vi "test.vi"() -> (0 "picture":picture)   [LabVIEW 2013]
uses:
  <vilib>/Analysis/NI_AALBase.lvlib
panel:
  in  "Size":cluster{"horz":i16, "vert":i16}
  out "Red":T1(graph)
  out "Blue":T1(graph)
  out "Green":T1(graph)
  out "Intensity Graph":u8[][](graph)
  in  "Rectangle":cluster{"left":i16, "top":i16}
  in  "path to JPEG file":path
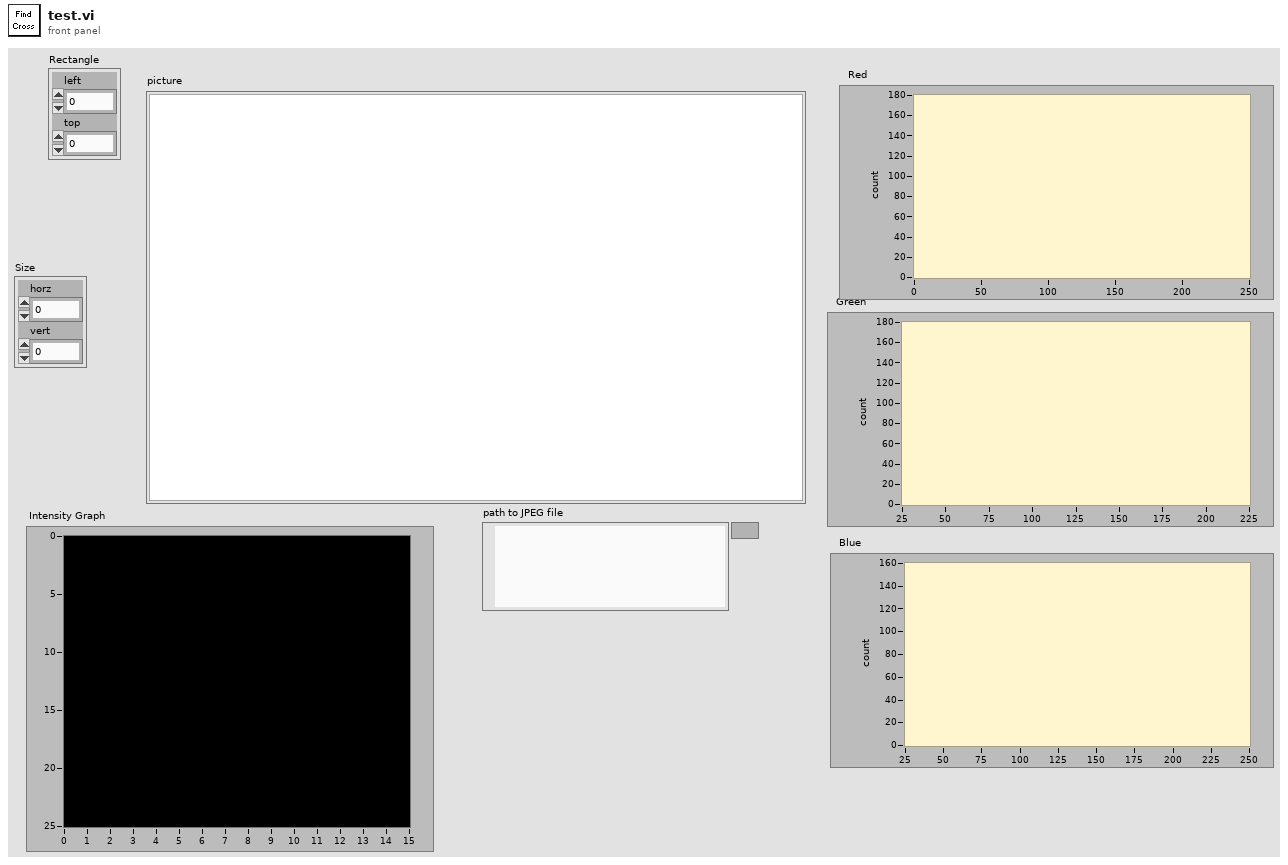
[diagram p1: front panel]
types:
  T1 = cluster{"X Values":dbl[], "Histogram: h(x)":i32[]}
  T2 = cluster{"left":i16, "top":i16, "right":i16, "bottom":i16}
  T3 = typedef "imagedata.ctl" = cluster{"image type":i32, "image depth":i32, "image":u8[], "mask":u8[], "colors":u32[], "Rectangle":cluster{"left":i16, "top":i16, "right":i16, "bottom":i16}}
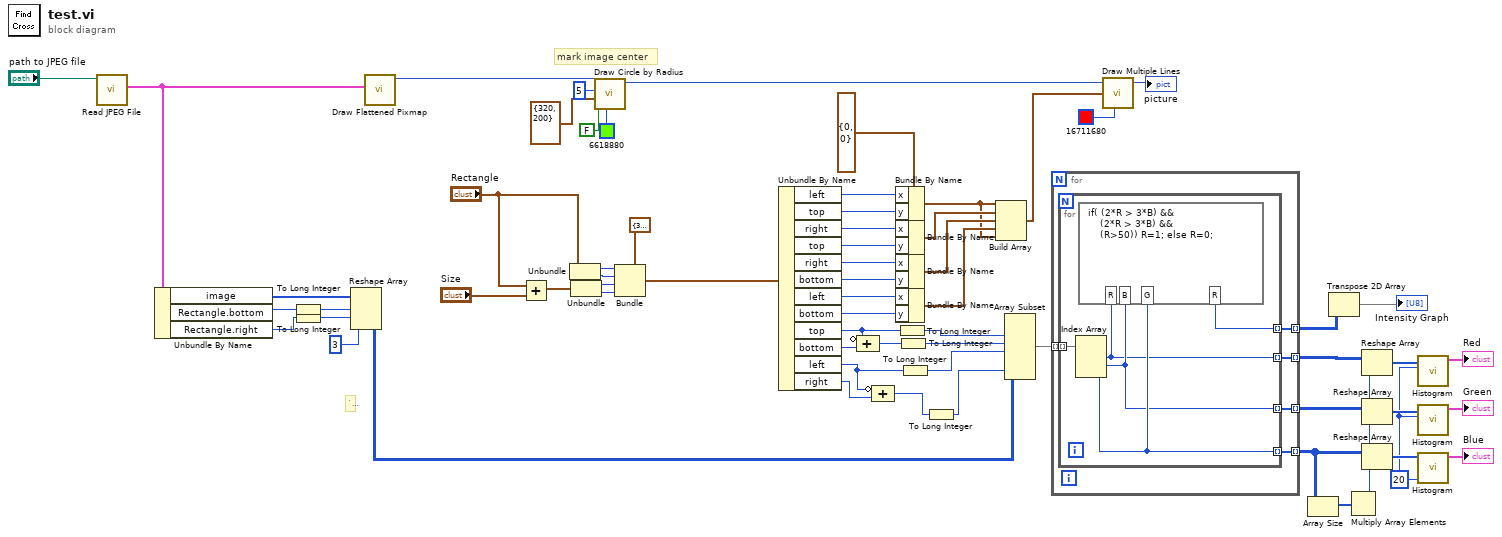
[diagram p0: block diagram]
diagram:
  w1 = 20 ("intervals")
  w55 = cluster{"x":i16, "y":i16} {"x"=0, "y"=0}
  # "``"
  # "mark image center"
  n1 = call <vilib>:"Read JPEG File.vi"("path to JPEG file"="path to JPEG file") -> ("image data"=w42:T3)  [unwired: 8 in, 2 out]
  n2 = Unbundle By Name(w42) -> ("image"=w41:u8[], "Rectangle.bottom"=w14:i16, "Rectangle.right"=w13:i16)
  n3 = To Long Integer(number=w14) -> (32bit integer=w12:i32)
  n4 = To Long Integer(number=w13) -> (32bit integer=w11:i32)
  n5 = Reshape Array(w41, w12, w11, 3 ("dimension size")) -> (w39:u8[][][])
  n6 = call <vilib>:"Draw Flattened Pixmap.vi"("image data"=w42) -> ("new picture"=w65:picture)  [unwired: 8 in]
  n7 = Add(x="Rectangle", y="Size") -> (x+y=w19:cluster{i16, i16})
  n8 = Unbundle("Rectangle") -> ("left"=w23:i16, "top"=w22:i16)
  n9 = Unbundle(w19) -> (w18:i16, w17:i16)
  n10 = call <vilib>:"Draw Circle by Radius.vi"("color(black)"=u32 6618880, "fill?(F)"=FALSE, "pixel center"=cluster{"horizontal":i16, "vertical":i16} {"horizontal"=320, "vertical"=200}, "radius"=i16 5, "picture"=w65) -> ("new picture"=w59:picture)  [unwired: 6 in]
  n11 = Bundle(cluster=T2 {"left"=300, "top"=100, "right"=400, "bottom"=200} ("Rectangle"), "left"=w23, "top"=w22, "right"=w18, "bottom"=w17) -> (w16:T2)
  n12 = Unbundle By Name(w16) -> ("left"=w57:i16, "top"=w56:i16, "right"=w54:i16, "top"=w53:i16, "right"=w52:i16, "bottom"=w51:i16, "left"=w50:i16, "bottom"=w49:i16, "top"=w8:i16, "bottom"=w9:i16, "left"=w7:i16, "right"=w6:i16)
  n13 = Compound Arithmetic op=ADD(invert w8, w9) -> (w37:i16)
  n14 = Compound Arithmetic op=ADD(invert w7, w6) -> (w5:i16)
  n15 = Bundle By Name(cluster=w55, "x"=w57, "y"=w56) -> (w43:cluster{"x":i16, "y":i16})
  n16 = Bundle By Name(cluster=w55, "x"=w54, "y"=w53) -> (w48:cluster{"x":i16, "y":i16})
  n17 = Bundle By Name(cluster=w55, "x"=w52, "y"=w51) -> (w47:cluster{"x":i16, "y":i16})
  n18 = Bundle By Name(cluster=w55, "x"=w50, "y"=w49) -> (w46:cluster{"x":i16, "y":i16})
  n19 = To Long Integer(number=w8) -> (32bit integer=w38:i32)
  n20 = To Long Integer(number=w37) -> (32bit integer=w36:i32)
  n21 = To Long Integer(number=w7) -> (32bit integer=w35:i32)
  n22 = To Long Integer(number=w5) -> (32bit integer=w4:i32)
  n23 = Build Array(w43, w48, w47, w46, w43) -> (w45:cluster{"x":i16, "y":i16}[])
  n24 = Array Subset(array=w39, index (dim 0)=w38, length (dim 0)=w36, index (dim 1)=w35, length (dim 1)=w4) -> (w34:u8[][][])  [unwired: 2 in]
  n25 = for {
    tunnel: w34 -> [w70] mode=indexing
    tunnel: [w69] -> w2 mode=indexing
    tunnel: [w68] -> w32 mode=indexing
    tunnel: [w67] -> w10 mode=indexing
    tunnel: [w66] -> w3 mode=indexing
    n26 = for {
      tunnel: w70 -> [w75] mode=indexing
      tunnel: [w72] -> w69 mode=indexing
      tunnel: [w73] -> w68 mode=indexing
      tunnel: [w74] -> w67 mode=indexing
      tunnel: [w71] -> w66 mode=indexing
      n27 = Index Array(array=w75) -> (element #1=w72:u8, element #2=w73:u8, element #3=w74:u8)  [unwired: 3 in]
      n28 = formula code="if( (2*R > 3*B) &&\n    (2*R > 3*B) &&\n    (R>50)) R=1; else R=0;"("R"=w72, "B"=w73, "G"=w74) -> ("R"=w71:u8)
    }
  }
  n29 = call <vilib>:"Draw Multiple Lines.vi"("picture"=w59, "line endpoints"=w45, "color(black)"=u32 16711680) -> ("new picture"=→"picture":picture)  [unwired: 6 in]
  n30 = Array Size(array=w10) -> (size(s)=w31:i32[])
  n31 = Transpose 2D Array(2D array=w3) -> (transposed array=→"Intensity Graph":u8[][])
  n32 = Multiply Array Elements(1:w31) -> (0:w28:i32)
  n33 = Reshape Array(w2, w28) -> (w29:u8[])
  n34 = Reshape Array(w32, w28) -> (w33:u8[])
  n35 = Reshape Array(w10, w28) -> (w30:u8[])
  n36 = call <vilib>:"Histogram.vi"("intervals"=w1, "X"=w29) -> ("Histogram Graph"=→"Red":T1)  [unwired: 6 in, 3 out]
  n37 = call <vilib>:"Histogram.vi"("intervals"=w1, "X"=w33) -> ("Histogram Graph"=→"Green":T1)  [unwired: 6 in, 3 out]
  n38 = call <vilib>:"Histogram.vi"("intervals"=w1, "X"=w30) -> ("Histogram Graph"=→"Blue":T1)  [unwired: 6 in, 3 out]
